vi "Get Alarm Status.vi"(8 "error in":errorcluster, 11 "TE Cooler in":refnum<class "TE Cooler.lvclass">) -> (0 "error out":errorcluster, 2 "alarms":T1, 3 "TE Cooler out":refnum<class "TE Cooler.lvclass">)   [LabVIEW 2015, in "TE Cooler.lvlib" / "TE Cooler.lvclass"]
uses:
  TE Cooler.lvclass
  Controls/Command.ctl
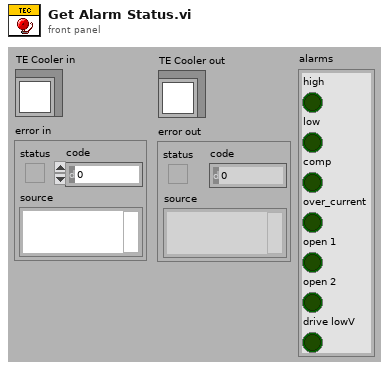
[diagram p1: front panel]
types:
  T1 = cluster{"high":bool, "low":bool, "comp":bool, "over_current":bool, "open 1":bool, "open 2":bool, "drive lowV":bool}
  T2 = typedef "TE Cooler.lvlib/TE Cooler.lvclass/Command.ctl" = enum16{"INPUT1", "DESIRED CONTROL VALUE", "POWER OUTPUT", "ALARM STATUS", "INPUT 2", "OUTPUT CURRENT COUNTS", "ALARM TYPE", "SET TYPE DEFINE", "SENSOR TYPE", "CONTROL TYPE", "CONTROL OUTPUT POLARITY", "POWER ON/OFF", "OUTPUT SHUTDOWN IF ALARM", "FIXED DESIRED CONTROL SETTING", "PROPORTIONAL BANDWIDTH", "INTEGRAL GAIN", "DERIVATIVE GAIN", "LOW EXTERNAL SET RANGE", "HIGH EXTERNAL SET RANGE", "ALARM DEADBAND", "HIGH ALARM SETTING", "LOW ALARM SETTING", "CONTROL DEADBAND SETTING", "INPUT1 OFFSET", "INPUT2 OFFSET", "HEAT MULTIPLIER", "COOL MULTIPLIER", "OVER CURRENT COUNT COMPARE VALUE", "ALARM LATCH ENABLE", "NOT USED", "ALARM LATCH RESET", "CHOOSE SENSOR FOR ALARM FUNCTION", "CHOOSE TEMPERATURE WORKING UNITS", "EEPROM WRITE ENABLE", "OVER CURRENT CONTINUOUS", "OVER CURRENT RESTART ATTEMPTS", "JP3 DISPLAY ENABLE"}
  T3 = cluster{"[0]":bool, "[1]":bool, "[2]":bool, "[3]":bool, "[4]":bool, "[5]":bool, "[6]":bool}
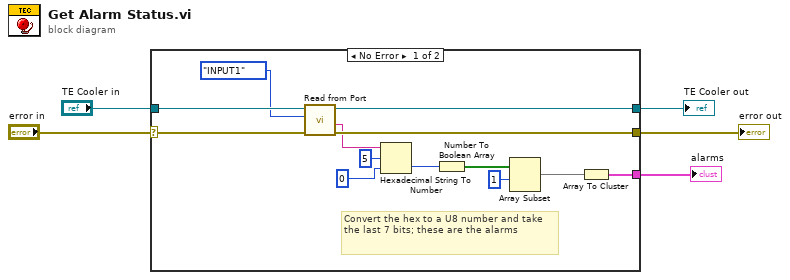
[diagram p0: block diagram]
diagram:
  n1 = case shown="No Error" "error in" {
    selector: "error in" -> [w17 w20]
    tunnel: [w15 w20] -> w4
    tunnel: [w16 w19] -> w2
    tunnel: "TE Cooler in" -> [w18 w19]
    tunnel: [w6 _] -> w1
    frame No Error {
      # "Convert the hex to a U8 number and take the last 7 bits; these are the alarms"
      n2 = call "Read from Port.vi"("error in"=w17, "TEC Cmd"=Command."INPUT1", "TE Cooler in"=w18) -> ("error out"=w15:errorcluster, "outputStr"=w13:string, "TE Cooler out"=w16:refnum<class "TE Cooler.lvclass">)  [unwired: 5 in, 1 out]
      n3 = Hexadecimal String To Number(string=w13, offset=5, default (0uL)=u8 0 ("default (0 U32)")) -> (number=w12:u8)  [unwired: 1 out]
      n4 = Number To Boolean Array(number=w12) -> (Boolean array=w9:bool[])
      n5 = Array Subset(array=w9, index=1) -> (w7:bool[])  [unwired: 1 in]
      n6 = Array To Cluster(array=w7) -> (cluster=w6:T3)
    }
    frame Error {
    }
  }
  "error out" <- w4
  "TE Cooler out" <- w2
  "alarms" <- w1
